vi "Read_PhotonVisionData.vi"() -> ()   [LabVIEW 2020]
uses:
  <vilib>/Rock Robotics/WPI/ThirdParty/PhotonVisionLib/TypeDef/PhotonPipelineResultType.ctl
  <vilib>/Rock Robotics/WPI/ThirdParty/PhotonVisionLib/TypeDef/PhotonTrackedTargetType.ctl
  <vilib>/Rock Robotics/WPI/ThirdParty/PhotonVisionLib/TypeDef/TargetCornerType.ctl
  <vilib>/Rock Robotics/WPI/ThirdParty/JAS_Junk/TrajLib/TypeDef/TRANSFORM3D.ctl
  <vilib>/Rock Robotics/WPI/ThirdParty/JAS_Junk/TrajLib/TypeDef/TRANSLATION3D.ctl
  <vilib>/Rock Robotics/WPI/ThirdParty/JAS_Junk/TrajLib/TypeDef/ROTATION3D.ctl
  <vilib>/Rock Robotics/WPI/ThirdParty/JAS_Junk/TrajLib/TypeDef/QUATERNION.ctl
  <vilib>/Rock Robotics/WPI/Utilities/WPI_GetSetVariantRefNum.vi
  <vilib>/Rock Robotics/Network Tables/NT Write Boolean.vi
  <vilib>/Rock Robotics/Network Tables/NT Write Number.vi
  <vilib>/Rock Robotics/WPI/ThirdParty/PhotonVisionLib/PhotonVisionLib.lvlib
  <vilib>/Rock Robotics/WPI/ThirdParty/JAS_Junk/TrajLib/Trajectory_Library.lvlib
panel:
  out "CtrlLibDistToBestTarg\nMeters":dbl
  out "Loop Count":i32
  out "SpecificPhotonTrackedTarget":T1={"Yaw"=0.0, "Pitch"=0.0, "Area"=0.0, "Skew"=0.0, "TargetCorners"=[], "BestCameraToTarget"={"TRANSLATION3D"={"X"=0.0, "Y"=0.0, "Z"=0.0}, "ROTATION3D"={"Q_quaternion"={"R"=1.0, "V"=[0.0, 0.0, 0.0]}}, "XF"=FALSE}, "FiiducialId"=0, "AltCameraToTarget"={"TRANSLATION3D"={"X"=0.0, "Y"=0.0, "Z"=0.0}, "ROTATION3D"={"Q_quaternion"={"R"=0.0, "V"=[0.0, 0.0, 0.0]}}, "XF"=FALSE}, "PoseAmbiguity"=0.0} {"AltCameraToTarget"."TRANSLATION3D"."Z" format="%14.3f"; "AltCameraToTarget"."TRANSLATION3D"."Y" format="%14.3f"; "AltCameraToTarget"."TRANSLATION3D"."X" format="%14.3f"; "BestCameraToTarget"."TRANSLATION3D"."Z" format="%14.3f"; "BestCameraToTarget"."TRANSLATION3D"."Y" format="%14.3f"; "BestCameraToTarget"."TRANSLATION3D"."X" format="%14.3f"}
  out "PipelineResult":T7 {"Targets"."AltCameraToTarget"."TRANSLATION3D"."Z" format="%14.3f"; "Targets"."AltCameraToTarget"."TRANSLATION3D"."Y" format="%14.3f"; "Targets"."AltCameraToTarget"."TRANSLATION3D"."X" format="%14.3f"; "Targets"."BestCameraToTarget"."TRANSLATION3D"."Z" format="%14.3f"; "Targets"."BestCameraToTarget"."TRANSLATION3D"."Y" format="%14.3f"; "Targets"."BestCameraToTarget"."TRANSLATION3D"."X" format="%14.3f"}
  out "SpecificTargetFound":bool
  out "TagTarget Index":i32
  in  "Fiiducial ID":i32
  out "BestTargetFound":bool
  out "BestYaw":dbl
  out "DistanceToBestTarget \nMeters":dbl
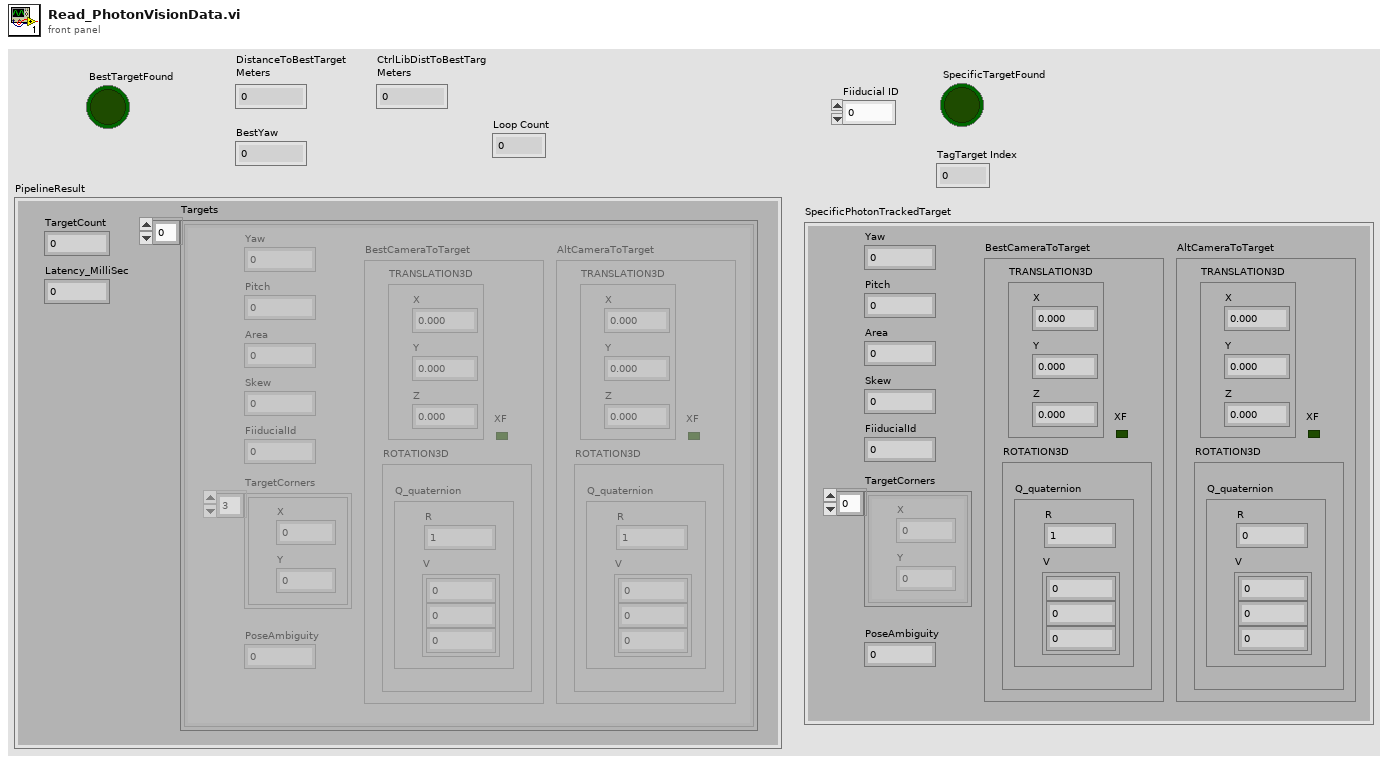
[diagram p1: front panel]
types:
  T1 = typedef "PhotonVisionLib.lvlib/PhotonTrackedTargetType.ctl" = cluster{"Yaw":dbl, "Pitch":dbl, "Area":dbl, "Skew":dbl, "TargetCorners":T2[], "BestCameraToTarget":T3, "FiiducialId":i32, "AltCameraToTarget":T3, "PoseAmbiguity":dbl}
  T2 = typedef "PhotonVisionLib.lvlib/TargetCornerType.ctl" = cluster{"X":dbl, "Y":dbl}
  T3 = typedef "Trajectory_Library.lvlib/TRANSFORM3D.ctl" = cluster{"TRANSLATION3D":T4, "ROTATION3D":T5, "XF":bool}
  T4 = typedef "Trajectory_Library.lvlib/TRANSLATION3D.ctl" = cluster{"X":dbl, "Y":dbl, "Z":dbl}
  T5 = typedef "Trajectory_Library.lvlib/ROTATION3D.ctl" = cluster{"Q_quaternion":T6}
  T6 = typedef "Trajectory_Library.lvlib/QUATERNION.ctl" = cluster{"R":dbl, "V":dbl[]}
  T7 = typedef "PhotonVisionLib.lvlib/PhotonPipelineResultType.ctl" = cluster{"TargetCount":i32, "Latency_MilliSec":dbl, "Targets":T1[]}
  T8 = typedef "WPI_RobotDriveDevRef.ctl" = cluster{"DevStatus":errorcluster, "Motors[]":T9[], "Square Inputs":bool, "Max Output":dbl}
  T9 = typedef "WPI_MotorControlDeviceRef.ctl" = cluster{"DeviceStatus":errorcluster, "Type":T10, "PWM":cluster{"PWM Channel":T11, "DeadBand":T12}, "CAN":cluster{"Device Number":u8, "SetOutput VI Ref":variant, "GetOutput VI Ref":variant, "Enable VI Ref":variant, "Disable VI Ref":variant, "Data":variant}, "Invert":bool, "DIO PWM":cluster{"PWM \"Enable\" Channel":T11, "DIOChannel":T13, "PWM Rate":dbl}}
  T10 = typedef "WPI_MotorControlType.ctl" = enum16{"PWM", "CAN", "DIO PWM"}
  T11 = typedef "FPGA_DIOPWMChannel.ctl" = enum8{"PWM 0", "PWM 1", "PWM 2", "PWM 3", "PWM 4", "PWM 5", "PWM 6", "PWM 7", "PWM 8", "PWM 9", "PWM MXP 0", "PWM MXP 1", "PWM MXP 2", "PWM MXP 3", "PWM MXP 4", "PWM MXP 5", "PWM MXP 6", "PWM MXP 7", "PWM MXP 8", "PWM MXP 9", "Invalid"}
  T12 = typedef "WPI_PWMDeadband.ctl" = cluster{"Name":string, "maxPositivePwm":i32, "minPositivePwm":i32, "centerPwm":i32, "maxNegativePwm":i32, "minNegativePwm":i32, "angularRange":u16}
  T13 = typedef "FPGA_DIOChannel.ctl" = enum8{"DIO 0", "DIO 1", "DIO 2", "DIO 3", "DIO 4", "DIO 5", "DIO 6", "DIO 7", "DIO 8", "DIO 9", "DIO MXP 0", "DIO MXP 1", "DIO MXP 2", "DIO MXP 3", "DIO MXP 4", "DIO MXP 5", "DIO MXP 6", "DIO MXP 7", "DIO MXP 8", "DIO MXP 9", "DIO MXP 10", "DIO MXP 11", "DIO MXP 12", "DIO MXP 13", "DIO MXP 14", "DIO MXP 15", "SPI Port CS1", "SPI Port CS2", "SPI Port CS3", "SPI Port MISO", "SPI Port MOSI", "Invalid"}
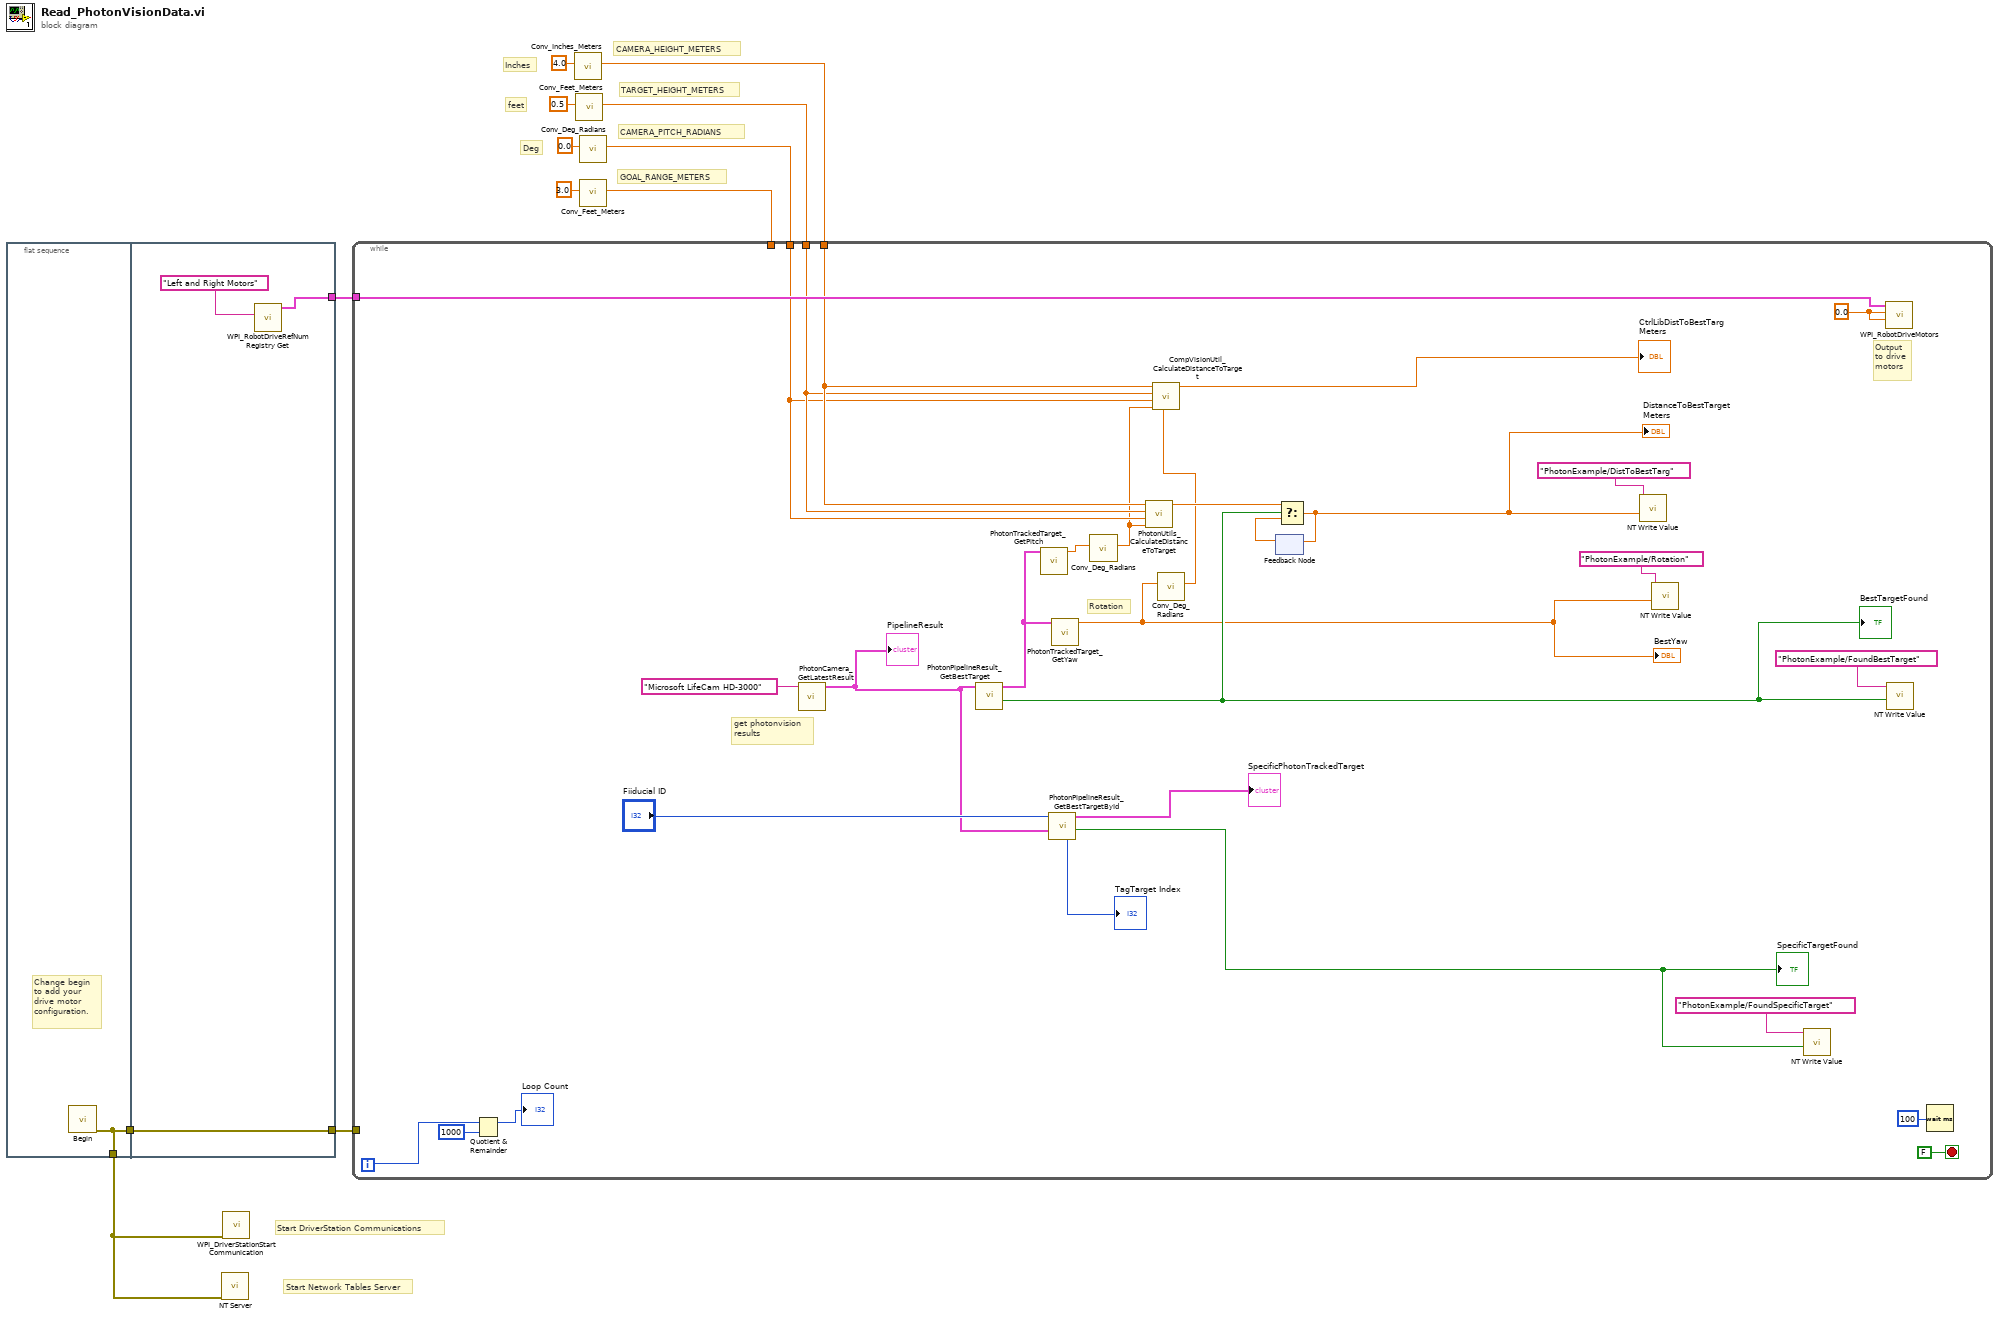
[diagram p0: block diagram]
diagram:
  # "Deg"
  # "feet"
  # "Inches"
  # "GOAL_RANGE_METERS"
  # "CAMERA_PITCH_RADIANS"
  # "TARGET_HEIGHT_METERS"
  # "CAMERA_HEIGHT_METERS"
  # "Start Network Tables Server"
  # "Start DriverStation Communications"
  n1 = flat-sequence {
    tunnel: [w13] -> w12
    tunnel: [w13] -> w2
    tunnel: [w16] -> w3
    tunnel: w2 -> [w16]
    tunnel: [w14] -> w1
    frame #0 {
      # "Change begin\nto add your \ndrive motor\nconfiguration."
      n2 = call "Begin.vi"() -> ("error out"=w13:errorcluster)  [unwired: 11 in]
    }
    frame #1 {
      n3 = call <vilib>:"WPI_RobotDriveRefNum Registry Get.vi"("refnum name"="Left and Right Motors") -> ("RobotDriveDevRef"=w14:T8)  [unwired: 9 in, 1 out]
    }
  }
  n4 = call <vilib>:"NT Server.vi"("error in (no error)"=w12) -> ()  [unwired: 11 in]
  n5 = call <vilib>:"WPI_DriverStationStart Communication.vi"("error in (no error)"=w12) -> ()  [unwired: 11 in]
  n6 = call <vilib>:"Conv_Inches_Meters.vi"("INCH"=4.0) -> ("Meters"=w7:dbl)  [unwired: 10 in]
  n7 = call <vilib>:"Conv_Feet_Meters.vi"("Feet"=0.5) -> ("Meters"=w6:dbl)  [unwired: 10 in]
  n8 = call <vilib>:"Conv_Feet_Meters.vi"("Feet"=3.0) -> ("Meters"=w4:dbl)  [unwired: 10 in]
  n9 = call <vilib>:"Conv_Deg_Radians.vi"("Degress"=0.0) -> ("Radians"=w5:dbl)  [unwired: 10 in]
  n10 = while {
    tunnel: w7 -> [w23]
    tunnel: w6 -> [w22]
    tunnel: w5 -> [w21]
    tunnel: w4 -> [_]
    tunnel: w3 -> [_]
    tunnel: w1 -> [w44]
    i -> [w26]
    stop <- FALSE stop-if-true
    w39 = 0.0 ("LeftSpeed")
    # "Rotation"
    # "get photonvision\nresults"
    # "Output\nto drive\nmotors"
    n11 = Quotient & Remainder(x=w26, y=1000) -> (x-y*floor(x/y)=→"Loop Count":i32)  [unwired: 1 out]
    n12 = call <vilib>:"PhotonCamera_GetLatestResult.vi"("CameraName"="Microsoft LifeCam HD-3000") -> ("PipelineResult"=w31:T7)  [unwired: 9 in, 1 out]
    "PipelineResult" <- w31
    n13 = call <vilib>:"PhotonPipelineResult_GetBestTarget.vi"("PhotonPipelineResult"=w31) -> ("TargetFound"=w35:bool, "PhotonTrackedTarget"=w32:T1)  [unwired: 9 in]
    "BestTargetFound" <- w35
    n14 = call <vilib>:"PhotonTrackedTarget_GetPitch.vi"("TrackedTarget"=w32) -> ("Pitch"=w34:dbl)  [unwired: 10 in]
    n15 = call <vilib>:"PhotonPipelineResult_GetBestTargetById.vi"("PhotonPipelineResult"=w31, "FiducialId"="Fiiducial ID") -> ("Target Found"=w28:bool, "PhotonTrackedTarget"=→"SpecificPhotonTrackedTarget":T1, "Target Index"=→"TagTarget Index":i32)  [unwired: 7 in]
    "SpecificTargetFound" <- w28
    n16 = call <vilib>:"PhotonTrackedTarget_GetYaw.vi"("TrackedTarget"=w32) -> ("Yaw"=w19:dbl)  [unwired: 10 in]
    "BestYaw" <- w19
    n17 = call <vilib>:"Conv_Deg_Radians.vi"("Degress"=w34) -> ("Radians"=w20:dbl)  [unwired: 10 in]
    n18 = call <vilib>:"PhotonUtils_CalculateDistanceToTarget.vi"("TargetPitch_Radians"=w20, "CameraPitch_Radians"=w21, "TargetHeight_Meters"=w22, "CameraHeight_Meters"=w23) -> ("DistanceToTarget_Meters"=w38:dbl)  [unwired: 7 in]
    n19 = call <vilib>:"Conv_Deg_Radians.vi"("Degress"=w19) -> ("Radians"=w18:dbl)  [unwired: 10 in]
    n20 = call <vilib>:"CompVisionUtil_CalculateDistanceToTarget.vi"("TargetYawRadians"=w18, "targetPitch_Radians"=w20, "cameraPitch_Radians"=w21, "targetHeight_Meters"=w22, "cameraHeight_Meters"=w23) -> ("DistanceToTarget_Meters"=→"CtrlLibDistToBestTarg\nMeters":dbl)  [unwired: 6 in]
    n21 = feedback #1() -> (w36:dbl)  [unwired: 1 in]
    n22 = Select(t=w38, s=w35, f=w36) -> (s? t:f=w37:dbl)
    "DistanceToBestTarget \nMeters" <- w37
    n23 = feedback-in #1(w37) -> ()
    n24 = call-poly <vilib>:"NT Write Value.vi"("Numeric"=w37, "Name"="PhotonExample/DistToBestTarg") -> ()  [unwired: 9 in, 1 out]
    n25 = call-poly <vilib>:"NT Write Value.vi"("Numeric"=w19, "Name"="PhotonExample/Rotation") -> ()  [unwired: 9 in, 1 out]
    n26 = call-poly <vilib>:"NT Write Value.vi"("Boolean"=w28, "Name"="PhotonExample/FoundSpecificTarget") -> ()  [unwired: 9 in, 1 out]
    n27 = call <vilib>:"WPI_RobotDriveMotors.vi"("RightSpeed"=w39, "LeftSpeed"=w39, "RobotDriveDevRef"=w44) -> ()  [unwired: 6 in, 3 out]
    n28 = call-poly <vilib>:"NT Write Value.vi"("Boolean"=w35, "Name"="PhotonExample/FoundBestTarget") -> ()  [unwired: 9 in, 1 out]
    n29 = Wait (ms)(milliseconds to wait=u32 100) -> ()  [unwired: 1 out]
  }
